vi "1D Inverse DCT.vi"(11 "DCT {X}":dbl[](array[numeric])) -> (0 "error":i32, 3 "X":dbl[](array[numeric]))   [LabVIEW 2017, in "NI_AALPro.lvlib"]
doc: "Computes the inverse Discrete Cosine Transform (DCT) of the input sequence <B>DCT {X}</B>. Wire data to the <B>DCT {X}</B> input to determine the polymorphic instance to use or manually select the instance."
uses:
  NI_AALPro.lvlib
  lvanlys.dll
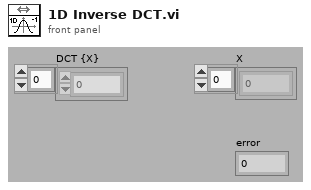
[diagram p1: front panel]
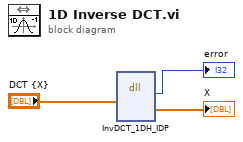
[diagram p0: block diagram]
diagram:
  n1 = dll-call lib="C:/Program Files/National Instruments/LabVIEW 2017/resource/lvanlys.*" fn="InvDCT_1DH_IDP"("xH"="DCT {X}") -> ("return type"=→"error":i32, "yH"=→"X":dbl[])  [unwired: 7 in, 2 out]
